vi "Plot Trajectory.vi"(11 "states":T1[](array[typedef])) -> (2 "Position":cluster{dbl[], dbl[]}(graph), 3 "Telemetry":cluster{dbl[], dbl[]}[](graph))   [LabVIEW 2019]
uses:
  Typedef/Trajectory State.ctl
  Geometry/Typedef/Pose2d.ctl
  Geometry/Typedef/Translation2d.ctl
  Geometry/Typedef/Rotation2d.ctl
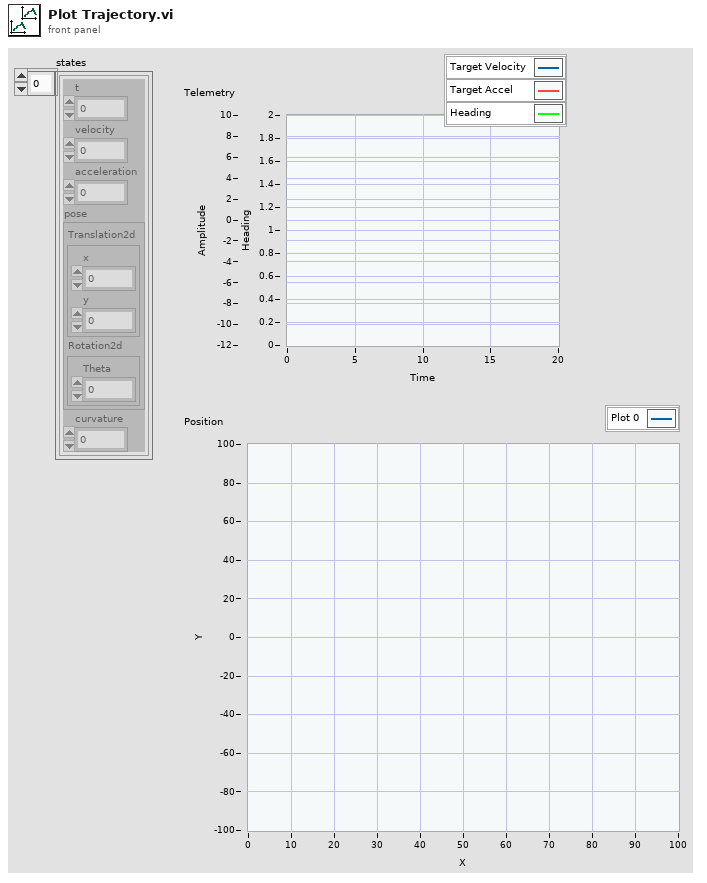
[diagram p1: front panel]
types:
  T1 = typedef "Trajectory State.ctl" = cluster{"t":dbl, "velocity":dbl, "acceleration":dbl, "pose":T2, "curvature":dbl}
  T2 = typedef "Pose2d.ctl" = cluster{"Translation2d":T3, "Rotation2d":T4}
  T3 = typedef "Translation2d.ctl" = cluster{"x":dbl, "y":dbl}
  T4 = typedef "Rotation2d.ctl" = cluster{"Theta":dbl}
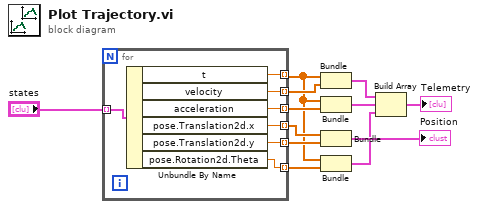
[diagram p0: block diagram]
diagram:
  n1 = for {
    tunnel: "states" -> [w19] mode=indexing
    tunnel: [w18] -> w3 mode=indexing
    tunnel: [w17] -> w5 mode=indexing
    tunnel: [w16] -> w6 mode=indexing
    tunnel: [w15] -> w11 mode=indexing
    tunnel: [w14] -> w10 mode=indexing
    tunnel: [w13] -> w2 mode=indexing
    n2 = Unbundle By Name(w19) -> ("t"=w18:dbl, "velocity"=w17:dbl, "acceleration"=w16:dbl, "pose.Translation2d.x"=w15:dbl, "pose.Translation2d.y"=w14:dbl, "pose.Rotation2d.Theta"=w13:dbl)
  }
  n3 = Bundle(w3, w5) -> (w7:cluster{dbl[], dbl[]})  [unwired: 1 in]
  n4 = Bundle(w3, w6) -> (w8:cluster{dbl[], dbl[]})  [unwired: 1 in]
  n5 = Bundle(w11, w10) -> (→"Position":cluster{dbl[], dbl[]})  [unwired: 1 in]
  n6 = Bundle(w3, w2) -> (w1:cluster{dbl[], dbl[]})  [unwired: 1 in]
  n7 = Build Array(w7, w8, w1) -> (→"Telemetry":cluster{dbl[], dbl[]}[])
